vi "FGV wait for 6 eMICs.vi"(7 "Enum":enum16{"Init", "count"}(ring), 8 "error in (no error)":errorcluster) -> (0 "error out":errorcluster, 2 "wait done":bool, 3 "count":u8)   [LabVIEW 2018, in "Application.lvlib"]
uses:
  Application.lvlib
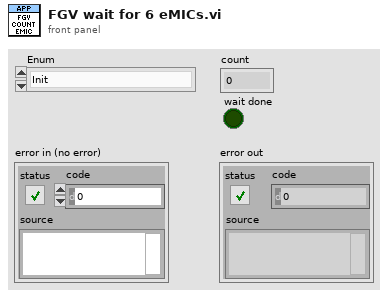
[diagram p1: front panel]
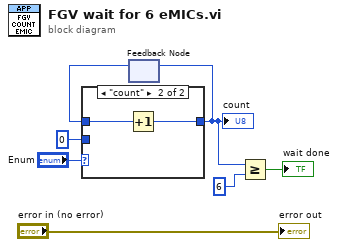
[diagram p0: block diagram]
diagram:
  n1 = feedback #1() -> (w5:u8)  [unwired: 1 in]
  n2 = case shown="\"count\"" "Enum" {
    tunnel: u8 0 -> [w8 _]
    tunnel: [w8 w9] -> w4
    tunnel: w5 -> [_ w10]
    frame "Init", Default {
    }
    frame "count" {
      n3 = Increment(x=w10) -> (x+1=w9:u8)
    }
  }
  "count" <- w4
  n4 = feedback-in #1(w4) -> ()
  n5 = Greater Or Equal?(x=w4, y=u8 6) -> (x >= y?=→"wait done":bool)
  "error out" <- "error in (no error)"
